vi "Leading Path Element Type.vi"(9 "error in (no error)":errorcluster, 11 "Path":string) -> (1 "error out":errorcluster, 2 "Path Element Type":T1)   [LabVIEW 2017, in "JSONtext.lvlib"]
uses:
  JSONtext.lvlib
  Parsing State.ctl
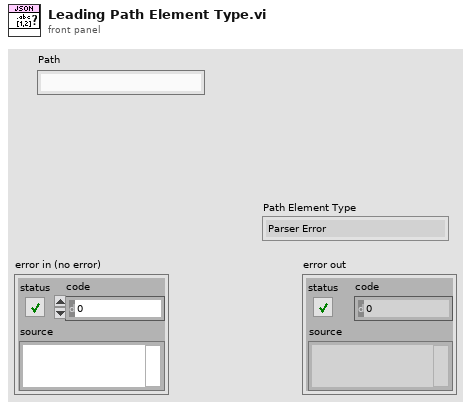
[diagram p1: front panel]
types:
  T1 = typedef "JSONtext.lvlib/Parsing State.ctl" = enum16{"Parser Error", "Object", "Array", "String", "Number/Other", "Leading Whitespace", "Object end", "Array end", "Value end"}
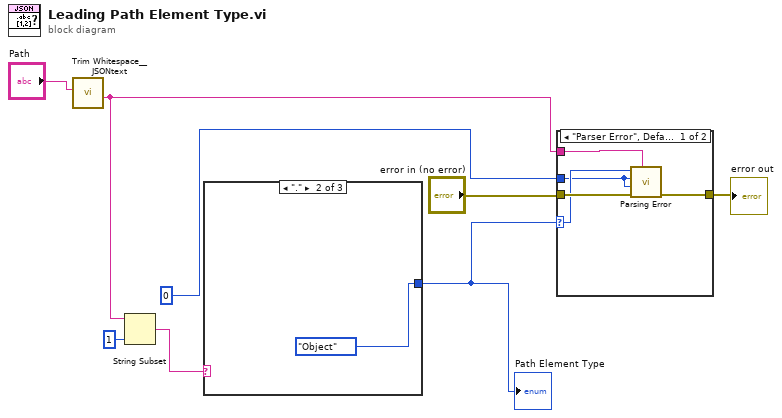
[diagram p0: block diagram]
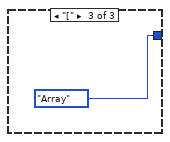
[diagram p3: hidden frame]
diagram:
  n1 = call "Trim Whitespace__JSONtext.vi"("String in"="Path") -> ("String out"=w5:string)  [unwired: 6 in]
  n2 = String Subset(string=w5, length (rest)=1 ("length (rest)")) -> (substring=w2:string)  [unwired: 1 in]
  n3 = case shown="\".\"" w2 {
    tunnel: [_ Parsing_State."Object" ("Parser State") Parsing_State."Array" ("Parser State")] -> w1
    frame Default {
    }
    frame "." {
    }
    frame "[" {
    }
  }
  "Path Element Type" <- w1
  n4 = case shown="\"Parser Error\", Default" w1 {
    selector: w1 -> [w12 _]
    tunnel: w5 -> [w15 _]
    tunnel: "error in (no error)" -> [w14 w16]
    tunnel: [w13 w16] -> w7
    tunnel: 0 -> [w11 _]
    frame "Parser Error", Default {
      n5 = call "Parsing Error.vi"("JSON"=w15, "error in (no error)"=w14, "Offset past match"=w11, "Value start"=w11, "State"=w12) -> ("error out"=w13:errorcluster)  [unwired: 6 in]
    }
    frame "Object", "Array" {
    }
  }
  "error out" <- w7
